vi "Read Inputs from system.vi"(8 "error in":errorcluster, 11 "MotionModule runtime in":refnum<class "MotionModule runtime.lvclass">) -> (0 "error out":errorcluster, 2 "Inputs from system":T1, 3 "MotionModule runtime out":refnum<class "MotionModule runtime.lvclass">)   [LabVIEW 2017, in "MotionModule runtime.lvclass"]
uses:
  MotionModule runtime.lvclass
  configuration/input data indices.ctl
  MotionModule runtime.lvclass/MotionModule runtime.ctl
  configuration/MotionModule configuration.lvclass
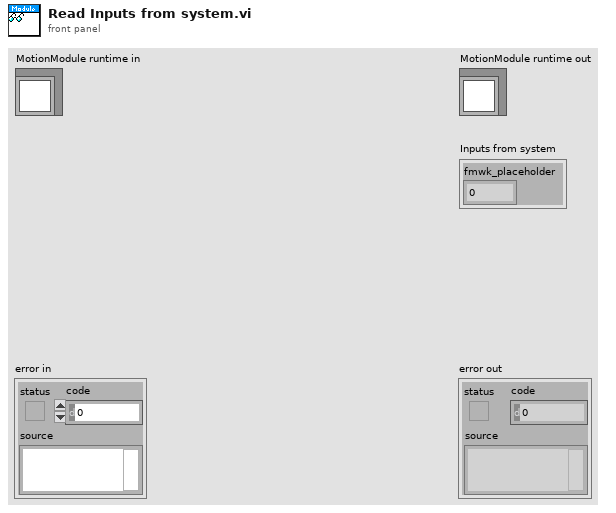
[diagram p1: front panel]
types:
  T1 = typedef "MotionModule configuration.lvclass/input data indices.ctl" = cluster{"fmwk_placeholder":i32}
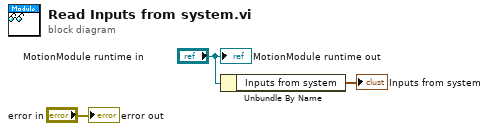
[diagram p0: block diagram]
diagram:
  n1 = Unbundle By Name("MotionModule runtime in") -> ("Inputs from system"=→"Inputs from system":T1)
  "error out" <- "error in"
  "MotionModule runtime out" <- "MotionModule runtime in"
